vi "HFRR ADV v024 new software.vi"() -> ()   [LabVIEW 2025] (continued)
                  }
                }
              }
            }
          }
        }
        n2655 = case shown="True" w3170 {
          frame False {
            n2656 = local write "tfalg"(0.0 ("tfalg")) -> ()
          }
          frame True {
            n2657 = local read "tfalg"() -> (w3315:dbl)
            n2658 = Equal?(x=w3315, y=0.0) -> (x = y?=w3316:bool)
            n2659 = case shown="True" w3316 {
              frame False {
              }
              frame True {
                n2660 = local read "Total No. of Tests"() -> (w3319:dbl)
                n2661 = local write "tfalg"(1.0 ("tfalg")) -> ()
                n2662 = local write "acq 2"(FALSE ("acq 2")) -> ()
                n2663 = Wait (ms)(milliseconds to wait=u32 200) -> ()  [unwired: 1 out]
                n2664 = Increment(x=w3319) -> (x+1=w3318:dbl)
                n2665 = local write "Total No. of Tests"(w3318) -> ()
              }
            }
          }
        }
        n2666 = local write "Test \nStatus"(w3176) -> ()
        n2667 = local write "Save"(w3176) -> ()
        n2668 = local read "Main Tab"() -> (w3133:T2)
        n2669 = case shown="True" w3157 {
          tunnel: [FALSE ("RUN") TRUE ("RUN")] -> w3156
          tunnel: [_ 1] -> w3149
          frame False {
          }
          frame True {
          }
        }
        n2670 = In Range and Coerce(upper limit=w3164, x=w3137, lower limit=w3163) -> (In Range?=w3155:bool)  [unwired: 1 out]
        n2671 = In Range and Coerce(upper limit=w3161, x=w3136, lower limit=w3162) -> (In Range?=w3153:bool)  [unwired: 1 out]
        n2672 = case shown="True" w3169 {
          frame False {
            n2673 = local read "Rt 3"() -> (w3297:bool)
            n2674 = case shown="True" w3297 {
              frame False {
              }
              frame True {
                n2675 = local write "Rt 3"(FALSE ("Rt 3")) -> ()
                n2676 = local write "Json End Flg"(TRUE ("Upld AR 2")) -> ()
              }
            }
            "Rt" <- TRUE ("Rt")
            "Rt 2" <- FALSE ("Rt")
          }
          frame True {
            n2677 = local read "Rt"() -> (w3304:bool)
            n2678 = local write "Rt 2"(TRUE ("Rt 2")) -> ()
            n2679 = case shown="True" w3304 {
              frame False {
              }
              frame True {
                w3305 = TRUE ("Upld AR 2")
                n2680 = local write "Rt"(FALSE ("Rt")) -> ()
                n2681 = local write "Upld AR"(w3305) -> ()
                n2682 = local write "Json St Flg"(w3305) -> ()
              }
            }
            "Rt 3" <- TRUE ("Rt 3")
          }
        }
        n2683 = case shown="True" w3155 {
          tunnel: [FALSE ("RUN") TRUE ("RUN")] -> w3154
          tunnel: [_ 2] -> w3148
          frame False {
          }
          frame True {
          }
        }
        n2684 = case shown="True" w3153 {
          tunnel: [FALSE ("RUN") TRUE ("RUN")] -> w3152
          tunnel: [_ 3] -> w3147
          frame False {
          }
          frame True {
          }
        }
        n2685 = case shown="\"Acquire\"" w3133 {
          tunnel: w3135 -> [_ w3366]
          frame Default {
            w3365 = 0.0 ("output")
            n2686 = local write "PID-out"(w3365) -> ()
            n2687 = local write "Frequency ( Hz )"(w3365) -> ()
          }
          frame "Acquire" {
            n2688 = stacked-sequence {
              frame #0 {
                n2689 = local read "Auto Start Test"() -> (w3368:bool)
                n2690 = case shown="True" w3368 {
                  tunnel: "RUN" -> [w3389 w3392]
                  tunnel: [w3389 w3391] -> w3369
                  frame False {
                  }
                  frame True {
                    n2691 = local read "Auto Start Temp"() -> (w3390:bool)
                    n2692 = Or(x=w3392, y=w3390) -> (x .or. y?=w3391:bool)
                  }
                }
                n2693 = local read "clk"() -> (w3388:dbl)
                n2694 = local read "Save"() -> (w3384:bool)
                n2695 = Equal?(x=w3388, y=0.0) -> (x = y?=w3385:bool)
                n2696 = And(x=w3385, y=w3384) -> (x .and. y?=w3386:bool)
                n2697 = Not(x="Engage") -> (.not. x?=w3375:bool)
                n2698 = case shown="False" w3369 {
                  tunnel: [0.0 w3415] -> w3371
                  frame False {
                    (unwired) TRUE ("Visible")
                    n2699 = local read "Auto Start Test"() -> (w3396:bool)
                    n2700 = local write "Start Time"(TRUE ("Start Time")) -> ()
                    n2701 = property on="Stroke 2" class="DigNum (strict)"("Visible"=FALSE) -> ()  [unwired: 2 in, 2 out]
                    n2702 = case shown="False" w3396 {
                      frame False {
                        n2703 = property on="Heater Button" class="Bool (strict)"("DisabledEnum"=T19."Enabled" ("Disabled")) -> ()  [unwired: 2 in, 2 out]
                        n2704 = property on="Humidity" class="Bool (strict)"("DisabledEnum"=T19."Enabled" ("Disabled")) -> ()  [unwired: 2 in, 2 out]
                      }
                      frame True {
                      }
                    }
                    n2705 = case shown="False" "TestCompFlg" {
                      frame False {
                        n2706 = local read "StartFlg"() -> (w3404:bool)
                        n2707 = case shown="True" w3404 {
                          frame False {
                          }
                          frame True {
                            n2708 = stacked-sequence {
                              frame #0 {
                                n2709 = local read "EVENT LOG"() -> (w3408:string)
                                n2710 = call "Event Log.vi"("Content"="Test was interrupted", "EVENT LOG"=w3408) -> ("EVENT LOG"=w3409:string)  [unwired: 8 in, 1 out]
                                n2711 = local write "EVENT LOG"(w3409) -> ()
                                n2712 = property on="RUN" class="Bool (strict)"("Visible"=TRUE) -> ()  [unwired: 2 in, 2 out]
                                n2713 = property on="Auto Start Test" class="Bool (strict)"("Visible"=TRUE) -> ()  [unwired: 2 in, 2 out]
                              }
                              frame #1 {
                                w3411 = FALSE ("StartFlg")
                                n2714 = property on="Heater Button" class="Bool (strict)"("Val(Sgnl)"=FALSE ("Value (Signaling)")) -> ()  [unwired: 2 in, 2 out]
                                n2715 = local write "Heater Button"(w3411) -> ()
                                n2716 = local write "StartFlg"(w3411) -> ()
                                n2717 = local write "Humidity"(w3411) -> ()
                              }
                              frame #2 {
                                n2718 = local write "Due Write"("VC;0" ("Command")) -> ()
                              }
                              frame #3 {
                                n2719 = Wait (ms)(milliseconds to wait=u32 1500) -> ()  [unwired: 1 out]
                              }
                              frame #4 {
                                n2720 = local write "Due Write"("HE;0" ("Command")) -> ()
                              }
                            }
                          }
                        }
                      }
                      frame True {
                      }
                    }
                    n2721 = local write "String 14"("Test will autostart once parameters reach the set value." ("String 14")) -> ()
                  }
                  frame True {
                    (unwired) FALSE ("Visible")
                    n2722 = property on="Stroke 2" class="DigNum (strict)"("Visible"=TRUE) -> ()  [unwired: 2 in, 2 out]
                    n2723 = property on="STOP 2" class="Bool (strict)"("Disabled"=u8 2) -> ()  [unwired: 2 in, 2 out]
                    n2724 = local write "String 14"(" Running....." ("String 14")) -> ()
                    n2725 = property on="Heater Button" class="Bool (strict)"("DisabledEnum"=T19."Disabled and Grayed Out" ("Disabled")) -> ()  [unwired: 2 in, 2 out]
                    n2726 = property on="Humidity" class="Bool (strict)"("DisabledEnum"=T19."Disabled and Grayed Out" ("Disabled")) -> ()  [unwired: 2 in, 2 out]
                    n2727 = case shown="True" "Start Time" {
                      selector: "Start Time" -> [_ w3434]
                      frame False {
                      }
                      frame True {
                        n2728 = Not(x=w3434) -> (.not. x?=w3433:bool)
                        n2729 = local write "Start Time"(w3433) -> ()
                        n2730 = local read "EVENT LOG"() -> (w3435:string)
                        n2731 = call "Event Log.vi"("Content"="Test in progress", "EVENT LOG"=w3435) -> ("EVENT LOG"=w3437:string)  [unwired: 8 in, 1 out]
                        n2732 = local write "EVENT LOG"(w3437) -> ()
                      }
                    }
                    n2733 = disable-structure shown="Enabled" {
                      disable-tunnel: [w3426 w3432] -> w3415
                      frame Disabled {
                        n2734 = local read "Set Hz"() -> (w3429:dbl)
                        n2735 = call <vilib>:"Uniform White Noise Waveform.vi"() -> ("signal out"=w3428:waveform(dbl))  [unwired: 10 in, 1 out]
                        n2736 = Random Number (0-1)() -> (number: 0 to 1=w3425:dbl)
                        n2737 = Add(x=w3429, y=w3428) -> (x+y=w3427:waveform(dbl))
                        n2738 = Multiply(x=ext 0.01 ("y"), y=w3425) -> (x*y=w3423:ext)
                        n2739 = Multiply(x=w3427, y=w3423) -> (x*y=w3426:waveform(ext))
                      }
                      frame Enabled {
                        n2740 = call-poly <vilib>:"Random Number (Range).vi"("lower bound (0)"=49.89, "upper bound (100)"=50.8) -> ("number"=w3432:dbl)  [unwired: 9 in]
                      }
                    }
                    "StartFlg" <- TRUE ("StartFlg")
                  }
                }
                n2741 = case shown="True" w3386 {
                  frame False {
                  }
                  frame True {
                    n2742 = local write "clk"(10.0 ("clk")) -> ()
                    n2743 = Get Date/Time In Seconds() -> (seconds since 1Jan1904=w3440:timestamp)
                    n2744 = To Double Precision Float(number=w3440) -> (double precision float=w3438:dbl)
                    n2745 = local write "acq timer"(w3438) -> ()
                    n2746 = local write "act save time"(w3438) -> ()
                  }
                }
                n2747 = call "Elapsed Time"("Time Target (s)"="Countdown", "Reset"=w3375) -> ("Elapsed Time (s)"=w3380:dbl, "Time has Elapsed"=w3378:bool)  [unwired: 10 in, 6 out]
                "Countdown 2" <- w3380
                n2748 = Subtract(x=w3380, y=2.0) -> (x-y=w3383:dbl)
                n2749 = Less?(x=w3383, y="Countdown") -> (x < y?=w3381:bool)
                n2750 = And(x=w3381, y=w3378) -> (x .and. y?=w3377:bool)
                n2751 = case shown="True" w3377 {
                  frame False {
                  }
                  frame True {
                    (unwired) dbl[] [] ("History Data")
                    n2752 = local write "Engage"(FALSE ("Engage")) -> ()
                    n2753 = local write "RUN"(TRUE ("RUN")) -> ()
                    n2754 = local read "Humidity ( %RH )"() -> (→"Rh Before":dbl)
                  }
                }
                n2755 = local read "Test \nStatus"() -> (w3373:bool)
                n2756 = Select(t=w3371, s=w3373, f=0.0) -> (s? t:f=w3372:dbl)
                n2757 = local write "Frequency ( Hz )"(w3372) -> ()
              }
              frame #1 {
                w3463 = 1000000.0 ("x")
                # "HC;1/0\nST;VALUE"
                # "Elapsed time\ncof\nstroke\nAir temp\nTemp\nHumidity"
                # "acq timer\n\nact save time"
                # "convert to microseconds"
                n2758 = local read "COUNT"() -> (w3446:i32)
                n2759 = local read "Rate"() -> (w3459:dbl)
                n2760 = Divide(x=w3463, y=w3459) -> (x/y=w3464:dbl)
                n2761 = Greater Or Equal?(x=w3446, y=250) -> (x >= y?=w3445:bool)
                n2762 = Get Date/Time In Seconds() -> (seconds since 1Jan1904=w3466:timestamp)
                n2763 = case shown="True" w3445 {
                  frame False {
                    n2764 = local read "COUNT"() -> (w3467:i32)
                    n2765 = Increment(x=w3467) -> (x+1=w3468:i32)
                    n2766 = local write "COUNT"(w3468) -> ()
                  }
                  frame True {
                    n2767 = local write "COUNT"(0 ("COUNT")) -> ()
                  }
                }
                n2768 = local read "Samplingtime 2"() -> (w3444:dbl)
                n2769 = local read "act save time"() -> (w3461:dbl)
                n2770 = Divide(x=w3464, y=w3463) -> (x/y=w3462:dbl)
                n2771 = To Double Precision Float(number=w3466) -> (double precision float=w3455:dbl)
                n2772 = Add(x=w3461, y=w3444) -> (x+y=w3460:dbl)
                n2773 = local read "acq timer"() -> (w3465:dbl)
                n2774 = local read "COUNT"() -> (w3448:i32)
                n2775 = Greater Or Equal?(x=w3455, y=w3460) -> (x >= y?=w3443:bool)
                n2776 = Multiply(x=w3462, y=w3448) -> (x*y=w3454:dbl)
                n2777 = Subtract(x=w3455, y=w3465) -> (x-y=w3457:dbl)
                n2778 = local read "Save"() -> (w3458:bool)
                n2779 = Add(x=w3457, y=w3454) -> (x+y=w3441:dbl)
                "Elapsed time 3" <- w3441
                n2780 = And(x=w3443, y=w3458) -> (x .and. y?=w3456:bool)
                n2781 = Divide(x=w3441, y=60.0) -> (x/y=w3452:dbl)
                n2782 = local read "Test \nStatus"() -> (w3442:bool)
                n2783 = local read "clk"() -> (w3449:dbl)
                n2784 = Equal?(x=w3449, y=10.0) -> (x = y?=w3451:bool)
                n2785 = case shown="True" w3456 {
                  tunnel: w3455 -> [_ w3579]
                  tunnel: [FALSE ("Boolean 2") TRUE ("Boolean 2")] -> _
                  frame False {
                  }
                  frame True {
                    w3533 = ";" ("Substring")
                    # "Pid out/\nFreq response value"
                    n2786 = local write "act save time"(w3579) -> ()
                    n2787 = local read "FILE"() -> (w3527:string)
                    n2788 = call "file check.vi"("file name in"=w3527) -> ("error out"=w3530:errorcluster, "file name out"=w3525:string)  [unwired: 9 in]
                    n2789 = local read "LVDT STROKE"() -> (w3522:dbl)
                    n2790 = local read "Add up Stroke"() -> (w3520:dbl)
                    n2791 = call "FILE PATH CREATION.vi"("error in"=w3530, "FILE NAME :"=w3525) -> ("FILE OUT"=w3528:path)  [unwired: 8 in, 1 out]
                    n2792 = Concatenate Strings(w3525, ".dgf" ("Substring")) -> (w3529:string)
                    n2793 = Subtract(x=w3522, y=w3520) -> (x-y=w3521:dbl)
                    n2794 = Absolute Value(x=w3521) -> (abs(x)=w3519:dbl)
                    n2795 = local read "FF 2"() -> (→"Frictional Force ( N )" →"Frictional Force ( N )":dbl)
                    n2796 = Build Path(base path=w3528, name or relative path=w3529) -> (appended path=w3524:path)
                    n2797 = local read "COF 2"() -> (w3538:dbl)
                    "cof" <- w3538
                    "Coefficient of Friction" <- w3538
                    "COF 4" <- w3538
                    "Coefficient of Friction" <- w3538
                    n2798 = local read "TEMP"() -> (w3541:dbl)
                    "Temp" <- w3541
                    "Temperature ( Deg C )" <- w3541
                    n2799 = local read "Humidity ( %RH )"() -> (w3540:dbl)
                    "Humidity ( %RH )" <- w3540
                    "Humidity ( %RH )" <- w3540
                    n2800 = local read "Frequency ( Hz )"() -> (w3547:dbl)
                    n2801 = call <vilib>:"Mean PtByPt.vi"("x"=w3519, "sample length"="STROKE FILTER") -> ("mean"=w3518:dbl)  [unwired: 2 in, 1 out]
                    n2802 = local read "Elapsed time"() -> (w3572:dbl)
                    n2803 = local read "AIR TEMP"() -> (w3545:dbl)
                    n2804 = local read "PID-out"() -> (w3550:dbl)
                    n2805 = local write "Temperature ( Deg C )"(w3541) -> ()
                    n2806 = Number To Fractional String(number=w3518, width (-)=i16 9 ("precision (6)"), precision (6)=i16 6) -> (F-format string=w3565:string)  [unwired: 1 in]
                    n2807 = Number To Fractional String(number=w3545, width (-)=i16 9 ("precision (6)"), precision (6)=i16 3) -> (F-format string=w3564:string)  [unwired: 1 in]
                    n2808 = Number To Fractional String(number=w3541, width (-)=i16 9 ("precision (6)"), precision (6)=i16 3) -> (F-format string=w3561:string)  [unwired: 1 in]
                    n2809 = Number To Fractional String(number=w3540, width (-)=i16 9 ("precision (6)"), precision (6)=i16 3) -> (F-format string=w3558:string)  [unwired: 1 in]
                    n2810 = Number To Fractional String(number=0.0, width (-)=i16 9 ("precision (6)"), precision (6)=i16 3) -> (F-format string=w3555:string)  [unwired: 1 in]
                    n2811 = Number To Fractional String(number=w3550, width (-)=i16 9 ("precision (6)"), precision (6)=i16 3) -> (F-format string=w3551:string)  [unwired: 1 in]
                    n2812 = Number To Fractional String(number=w3547, width (-)=i16 9 ("precision (6)"), precision (6)=i16 3) -> (F-format string=w3546:string)  [unwired: 1 in]
                    n2813 = Number To Fractional String(number=w3538, width (-)=i16 9 ("precision (6)"), precision (6)=i16 6) -> (F-format string=w3573:string)  [unwired: 1 in]
                    n2814 = Number To Fractional String(number=w3572, width (-)=i16 14 ("precision (6)"), precision (6)=i16 3) -> (F-format string=w3574:string)  [unwired: 1 in]
                    n2815 = Bundle("y"=1.02, "mean"=w3518, "y"=0.98) -> (w3539:cluster{"y":dbl, "mean":dbl, "y":dbl})  [unwired: 1 in]
                    n2816 = Number To Fractional String(number="Ambient Humidity :", width (-)=i16 9 ("precision (6)"), precision (6)=i16 6) -> (F-format string=w3531:string)  [unwired: 1 in]
                    n2817 = local read "RUN"() -> (w3537:bool)
                    n2818 = case shown="True" w3537 {
                      tunnel: w3539 -> [_ w3584]
                      tunnel: w3518 -> [_ w3583]
                      tunnel: w3518 -> [_ w3581]
                      tunnel: w3518 -> [_ w3582]
                      frame False {
                      }
                      frame True {
                        "Stroke ( mm )" <- w3584
                        "Stroke ( mm )" <- w3584
                        "Stroke 4" <- w3583
                        "Stroke 3" <- w3581
                        "Stroke 2" <- w3582
                        "measured_stroke" <- w3581
                      }
                    }
                    n2819 = Concatenate Strings(w3574, w3533, w3573, w3533, w3565, w3533, w3564, w3533, w3561, w3533, w3558, w3533, w3555, w3533, w3551, w3533, w3546, w3533, w3531, "\r") -> (w3571:string)
                    n2820 = call <vilib>:"Write Characters To File.vi"("append to file? (new file:F)"=TRUE, "character string"=w3571, "file path (dialog if empty)"=w3524) -> ()  [unwired: 2 in, 1 out]
                    "refresh flag" <- TRUE ("refresh flag")
                  }
                }
                n2821 = case shown="True" w3442 {
                  tunnel: w3452 -> [_ w3478]
                  tunnel: w3457 -> [_ w3488]
                  tunnel: [0.0 w3484] -> _
                  tunnel: w3451 -> [_ w3483]
                  tunnel: [0.0 w3482] -> _
                  tunnel: w3441 -> [_ w3482]
                  tunnel: w3455 -> [w3471 _]
                  frame False {
                    n2822 = local write "acq timer"(w3471) -> ()
                    n2823 = local write "Test Duration Status"(0.0 ("Test Duration Status")) -> ()
                  }
                  frame True {
                    n2824 = local read "Set Hz"() -> (w3485:dbl)
                    n2825 = local write "Elapsed time"(w3478) -> ()
                    n2826 = local read "test time"() -> (w3477:dbl)
                    n2827 = Multiply(x=w3488, y=w3485) -> (x*y=w3487:dbl)
                    n2828 = case shown="False" w3483 {
                      tunnel: w3487 -> [w3489 _]
                      tunnel: [w3489 1.0] -> w3484
                      frame False {
                        n2829 = local write "Cycles elapsed"(w3489) -> ()
                      }
                      frame True {
                      }
                    }
                    n2830 = Greater?(x=w3478, y=w3477) -> (0:w3486:bool)
                    n2831 = Subtract(x=w3477, y=w3478) -> (x-y=w3476:dbl)
                    "time" <- w3476
                    n2832 = Multiply(x=w3476, y=60.0) -> (x*y=w3475:dbl)
                    n2833 = local write "Time Remaining"(w3475) -> ()
                    n2834 = local write "Remaining Time"(w3475) -> ()
                    n2835 = case shown="True" w3486 {
                      frame False {
                      }
                      frame True {
                        n2836 = stacked-sequence {
                          frame #0 {
                            w3494 = T19."Enabled" ("Disabled")
                            w3493 = FALSE ("TEST FILE NAM,E SAVED")
                            w3495 = "" ("FILE")
                            w3496 = TRUE ("Visible")
                            n2837 = local write "Humidity"(FALSE ("Humidity")) -> ()
                            n2838 = local write "RUN"(FALSE ("OK Button 2")) -> ()
                            n2839 = local write "Heater Button"(FALSE ("Heater Button")) -> ()
                            n2840 = local write "Auto Start Test"(FALSE ("Auto Start Test")) -> ()
                            n2841 = local write "TestCompFlg"(TRUE ("StpFlg")) -> ()
                            n2842 = local read "Humidity ( %RH )"() -> (→"Rh After":dbl)
                            n2843 = property on="STOP 2" class="Bool (strict)"("Disabled"=u8 0) -> ()  [unwired: 2 in, 2 out]
                            n2844 = local read "EVENT LOG"() -> (w3501:string)
                            n2845 = call "Event Log.vi"("Content"="Test Completed", "EVENT LOG"=w3501) -> ("EVENT LOG"=w3500:string)  [unwired: 8 in, 1 out]
                            n2846 = property on="RUN" class="Bool (strict)"("Visible"=w3496) -> ()  [unwired: 2 in, 2 out]
                            n2847 = property on="Auto Start Test" class="Bool (strict)"("Visible"=w3496) -> ()  [unwired: 2 in, 2 out]
                            n2848 = local write "Batch Ref Num :"(w3495) -> ()
                            n2849 = local write "FILE"(w3495) -> ()
                            n2850 = local write "EVENT LOG"(w3500) -> ()
                            n2851 = local write "TEST FILE NAM,E SAVED"(w3493) -> ()
                            n2852 = local write "Fuel Discription :"(w3495) -> ()
                            n2853 = local write "START TEMP"(w3493) -> ()
                            n2854 = local write "Remarks :"(w3495) -> ()
                            n2855 = local write "Main Dashboard Buttons"(T1."Imaging" ("Main Dashboard Buttons")) -> ()
                            n2856 = local write "Main Tab"(T2."Adv Scar" ("Main Tab")) -> ()
                            n2857 = property on="FRICVALZ 2" class="Bool (strict)"("DisabledEnum"=w3494) -> ()  [unwired: 2 in, 2 out]
                            n2858 = property on="FRICVALZ 3" class="Bool (strict)"("DisabledEnum"=w3494) -> ()  [unwired: 2 in, 2 out]
                            n2859 = property on="FRICVALZ 4" class="Bool (strict)"("DisabledEnum"=w3494) -> ()  [unwired: 2 in, 2 out]
                          }
                          frame #1 {
                            n2860 = Wait (ms)(milliseconds to wait=u32 1500) -> ()  [unwired: 1 out]
                          }
                          frame #2 {
                            n2861 = local write "Due Write"("VC;0") -> ()
                          }
                          frame #3 {
                            n2862 = Wait (ms)(milliseconds to wait=u32 1500) -> ()  [unwired: 1 out]
                          }
                          frame #4 {
                            n2863 = local write "Due Write"("VC;0") -> ()
                          }
                          frame #5 {
                            n2864 = Wait (ms)(milliseconds to wait=u32 1500) -> ()  [unwired: 1 out]
                          }
                          frame #6 {
                            n2865 = local write "Due Write"("ST;0") -> ()
                          }
                          frame #7 {
                            n2866 = local write "measured_stroke"(0.0 ("measured_stroke")) -> ()
                            n2867 = Wait (ms)(milliseconds to wait=u32 1500) -> ()  [unwired: 1 out]
                          }
                          frame #8 {
                            n2868 = local write "Due Write"("HE;0") -> ()
                          }
                        }
                      }
                    }
                    n2869 = Divide(x=w3478, y=w3477) -> (x/y=w3481:dbl)
                    n2870 = Multiply(x=w3481, y=100.0) -> (x*y=w3479:dbl)
                    n2871 = local write "Test Duration Status"(w3479) -> ()
                  }
                }
              }
              frame #2 {
                n2872 = case shown="True" "Heater Button" {
                  tunnel: [0.0 ("output") w3607] -> w3585
                  frame False {
                    w3588 = TRUE ("tmpchk")
                    n2873 = local read "TEMP"() -> (w3589:dbl)
                    n2874 = local write "Temp ini"(w3589) -> ()
                    n2875 = local write "Reset 4"(w3588) -> ()
                    n2876 = local write "tmpchk"(w3588) -> ()
                    n2877 = local write "reinit"(TRUE ("reinit")) -> ()
                    n2878 = local write "manual temp log"(TRUE ("manual temp log")) -> ()
                  }
                  frame True {
                    # "Logic to turn off\nthe heater when \ntemp is not rising.\nTime - 60 sec\nDelta t- 5°c"
                    n2879 = local read "Temp ini"() -> (w3596:dbl)
                    n2880 = local read "Auto Start Test"() -> (w3592:bool)
                    n2881 = Less?(x=w3596, y=53.0) -> (x < y?=w3594:bool)
                    n2882 = case shown="False" w3592 {
                      frame False {
                        n2883 = local read "Set Temp"() -> (w3616:dbl)
                        n2884 = local read "TEMP"() -> (w3615:dbl)
                        n2885 = Subtract(x=w3616, y=w3615) -> (x-y=w3614:dbl)
                        n2886 = Absolute Value(x=w3614) -> (abs(x)=w3613:dbl)
                        n2887 = Less?(x=w3613, y=0.5) -> (x < y?=w3611:bool)
                        n2888 = case shown="True" w3611 {
                          tunnel: "manual temp log" -> [_ w3617]
                          frame False {
                          }
                          frame True {
                            n2889 = case shown="True" w3617 {
                              selector: w3617 -> [_ w3618]
                              frame False {
                              }
                              frame True {
                                # "#Event log"
                                n2890 = Not(x=w3618) -> (.not. x?=w3619:bool)
                                n2891 = local write "manual temp log"(w3619) -> ()
                                n2892 = local read "EVENT LOG"() -> (w3622:string)
                                n2893 = call "Event Log.vi"("Content"="Target Temperature reached", "EVENT LOG"=w3622) -> ("EVENT LOG"=w3621:string)  [unwired: 8 in, 1 out]
                                n2894 = local write "EVENT LOG"(w3621) -> ()
                              }
                            }
                          }
                        }
                      }
                      frame True {
                        n2895 = local write "manual temp log"(TRUE ("manual temp log")) -> ()
                      }
                    }
                    n2896 = And(x="tmpchk", y=w3594) -> (x .and. y?=w3597:bool)
                    n2897 = case shown="True" w3597 {
                      frame False {
                      }
                      frame True {
                        n2898 = call "Elapsed Time8"("Time Target (s)"=300.0, "Reset"="Reset 4") -> ("Time has Elapsed"=w3624:bool)  [unwired: 10 in, 7 out]
                        n2899 = flat-sequence {
                          tunnel: w3624 -> [_]
                          frame #0 {
                            n2900 = local write "Reset 4"(FALSE ("Reset 4")) -> ()
                          }
                        }
                        n2901 = case shown="True" w3624 {
                          frame False {
                          }
                          frame True {
                            n2902 = local read "Temp ini"() -> (w3631:dbl)
                            n2903 = Add(x=w3631, y=5.0) -> (x+y=w3629:dbl)
                            n2904 = local read "TEMP"() -> (w3632:dbl)
                            n2905 = Greater?(x=w3632, y=w3629) -> (0:w3630:bool)
                            n2906 = case shown="False" w3630 {
                              frame False {
                                n2907 = local write "Heater Button"(FALSE ("Heater Button")) -> ()
                              }
                              frame True {
                                n2908 = local write "tmpchk"(FALSE ("tmpchk")) -> ()
                              }
                            }
                          }
                        }
                      }
                    }
                    n2909 = local read "Set Temp"() -> (w3605:dbl)
                    n2910 = local read "TEMP"() -> (w3599:dbl)
                    n2911 = call-poly <vilib>:"PID.vi"("reinitialize? (F)"="reinit", "dt (s)"=-1.0, "process variable"=w3599, "setpoint"=w3605) -> ("output"=w3602:dbl)  [unwired: 6 in, 1 out]
                    n2912 = Subtract(x=w3605, y=w3599) -> (x-y=w3606:dbl)
                    n2913 = Add(x=w3605, y=0.5) -> (x+y=w3603:dbl)
                    n2914 = Greater Or Equal?(x=w3599, y=w3603) -> ()  [unwired: 1 out]
                    n2915 = Select(t=0.0, s=FALSE, f=w3602) -> (s? t:f=w3601:dbl)
                    "PID output" <- w3601
                    n2916 = flat-sequence {
                      tunnel: w3601 -> [w3635]
                      tunnel: [w3635] -> w3607
                      frame #0 {
                        n2917 = local write "reinit"(FALSE ("reinit")) -> ()
                      }
                    }
                    n2918 = Bundle(w3606, "output"=w3601, "TEMP"=w3599) -> ()  [unwired: 1 in, 1 out]
                  }
                }
                "PID-out" <- w3585
              }
              frame #3 {
                n2919 = local read "TEMP"() -> (w3637:dbl)
                n2920 = Greater Or Equal?(x=w3637, y="Set Temp 2") -> (x >= y?=w3642:bool)
                n2921 = case shown="True" w3642 {
                  tunnel: [FALSE TRUE] -> w3640
                  frame False {
                  }
                  frame True {
                  }
                }
                "Status 13" <- w3640
                n2922 = And(x=w3640, y="trip1 8") -> (x .and. y?=w3639:bool)
                n2923 = case shown="True" w3639 {
                  frame False {
                    n2924 = local write "Heater Trip Temp"(TRUE ("Heater Trip Temp")) -> ()
                  }
                  frame True {
                    w3645 = FALSE ("OK Button 2")
                    n2925 = case shown="True" "Heater Trip Temp" {
                      selector: "Heater Trip Temp" -> [_ w3647]
                      frame False {
                      }
                      frame True {
                        n2926 = Not(x=w3647) -> (.not. x?=w3646:bool)
                        n2927 = local read "EVENT LOG"() -> (w3650:string)
                        n2928 = local write "Heater Trip Temp"(w3646) -> ()
                        n2929 = call "Event Log.vi"("Content"="Heater Trip", "EVENT LOG"=w3650) -> ("EVENT LOG"=w3649:string)  [unwired: 8 in, 1 out]
                        n2930 = local write "EVENT LOG"(w3649) -> ()
                      }
                    }
                    n2931 = local write "RUN"(w3645) -> ()
                    n2932 = property on="Auto Start Test" class="Bool (strict)"("Value"=w3645) -> ()  [unwired: 2 in, 2 out]
                    n2933 = local write "Heater Button"(w3645) -> ()
                  }
                }
              }
            }
            n2934 = case shown="False" w3366 {
              frame False {
                n2935 = disable-structure shown="Disabled" {
                  frame Disabled {
                    n2936 = stacked-sequence {
                      frame #0 {
                        n2937 = local write "RUN"(FALSE ("OK Button 2")) -> ()
                      }
                      frame #1 {
                      }
                    }
                  }
                  frame Enabled {
                  }
                }
              }
              frame True {
              }
            }
          }
        }
        n2938 = local read "airtempflg"() -> (w3158:bool)
        n2939 = Or(x=w3158, y=w3156) -> (x .or. y?=w3159:bool)
        n2940 = Insert Into Array(array=string[] ["Air Temperature has reached set value,", "Humidity has reached set value,", "Sample Temperaturehas reached set value,", ""], index=0, new element="") -> (w3144:string[])
        n2941 = Build Array(w3149, w3148, w3147) -> (w3145:i32[])
        n2942 = disable-structure shown="Disabled" {
          disable-tunnel: w3159 -> [w3236 _]
          disable-tunnel: w3154 -> [w3235 _]
          disable-tunnel: w3152 -> [w3234 _]
          frame Disabled {
            n2943 = Compound Arithmetic op=AND(w3236, w3235, w3234) -> ()  [unwired: 1 out]
            n2944 = case shown="True" {
              selector: _ -> [_ _]
              frame False {
              }
              frame True {
                w3237 = FALSE ("autostrtflg")
                n2945 = local write "RUN"(TRUE ("RUN")) -> ()
                n2946 = local write "autostrtflg"(w3237) -> ()
                n2947 = local write "autostart"(w3237) -> ()
                n2948 = local write "String 14"(" Running....." ("String 14")) -> ()
              }
            }
          }
          frame Enabled {
          }
        }
        n2949 = for {
          tunnel: w3145 -> [w3287] mode=indexing
          tunnel: w3144 -> [w3286]
          shift-right: [w3283] -> w3143
          shift-left: "" -> [w3285]
          n2950 = Index Array(array=w3286, index=w3287) -> (element=w3284:string)
          n2951 = Concatenate Strings(w3284, w3285) -> (w3283:string)
        }
        n2952 = local write "autostart 2"(w3143) -> ()
        n2953 = local read "Reset Graph"() -> (w3132:bool)
        n2954 = case shown="True" w3132 {
          selector: w3132 -> [_ w3186]
          frame False {
          }
          frame True {
            w3200 = 0.0 ("X Scale.Range:Maximum")
            n2955 = Not(x=w3186) -> (.not. x?=w3185:bool)
            n2956 = local write "Reset Graph"(w3185) -> ()
            n2957 = property on="Electrical Contact Resistance ( % )" class="WFChart (strict)"("XScale.Maximum"=600.0 ("X Scale.Range:Maximum"), "XScale.Minimum"=0.0 ("X Scale.Range:Minimum"), "YScale.Maximum"=100.0 ("Y Scale.Range:Maximum"), "YScale.Minimum"=0.0 ("Y Scale.Range:Minimum")) -> ()  [unwired: 2 in, 2 out]
            n2958 = property on="Frictional Force ( N )" class="WFChart (strict)"("XScale.Maximum"=600.0 ("X Scale.Range:Maximum"), "XScale.Minimum"=0.0 ("X Scale.Range:Minimum"), "YScale.Maximum"=100.0 ("Y Scale.Range:Maximum"), "YScale.Minimum"=0.0 ("Y Scale.Range:Minimum")) -> ()  [unwired: 2 in, 2 out]
            n2959 = property on="Temperature ( Deg C )" class="WFChart (strict)"("XScale.Maximum"=600.0 ("X Scale.Range:Maximum"), "XScale.Minimum"=0.0 ("X Scale.Range:Minimum"), "YScale.Maximum"=100.0 ("Y Scale.Range:Maximum"), "YScale.Minimum"=0.0 ("Y Scale.Range:Minimum")) -> ()  [unwired: 2 in, 2 out]
            n2960 = property on="Humidity ( %RH )" class="WFChart (strict)"("XScale.Maximum"=600.0 ("X Scale.Range:Maximum"), "XScale.Minimum"=0.0 ("X Scale.Range:Minimum"), "YScale.Maximum"=100.0 ("Y Scale.Range:Maximum"), "YScale.Minimum"=0.0 ("Y Scale.Range:Minimum")) -> ()  [unwired: 2 in, 2 out]
            n2961 = property on="Stroke ( mm )" class="WFChart (strict)"("XScale.Maximum"=600.0 ("X Scale.Range:Maximum"), "XScale.Minimum"=0.0 ("X Scale.Range:Minimum"), "YScale.Maximum"=100.0 ("Y Scale.Range:Maximum"), "YScale.Minimum"=0.0 ("Y Scale.Range:Minimum")) -> ()  [unwired: 2 in, 2 out]
            n2962 = property on="Coefficient of Friction" class="WFChart (strict)"("XScale.Maximum"=600.0 ("X Scale.Range:Maximum"), "XScale.Minimum"=0.0 ("X Scale.Range:Minimum"), "YScale.Maximum"=100.0 ("Y Scale.Range:Maximum"), "YScale.Minimum"=0.0 ("Y Scale.Range:Minimum")) -> ()  [unwired: 2 in, 2 out]
            n2963 = property on="Electrical Contact Resistance ( % )" class="WFChart (strict)"("XScale.Minimum"=0.0 ("X Scale.Range:Minimum"), "XScale.Maximum"=600.0 ("X Scale.Range:Maximum"), "YScale.Minimum"=0.0 ("Y Scale.Range:Minimum"), "YScale.Maximum"=100.0 ("Y Scale.Range:Maximum")) -> ()  [unwired: 2 in, 2 out]
            n2964 = property on="Temperature ( Deg C )" class="WFChart (strict)"("XScale.Minimum"=0.0 ("X Scale.Range:Minimum"), "XScale.Maximum"=600.0 ("X Scale.Range:Maximum"), "YScale.Minimum"=0.0 ("Y Scale.Range:Minimum"), "YScale.Maximum"=100.0 ("Y Scale.Range:Maximum")) -> ()  [unwired: 2 in, 2 out]
            n2965 = property on="Coefficient of Friction" class="WFChart (strict)"("XScale.Minimum"=0.0 ("X Scale.Range:Minimum"), "XScale.Maximum"=600.0 ("X Scale.Range:Maximum"), "YScale.Maximum"=1.0 ("X Scale.Range:Minimum"), "YScale.Minimum"=0.0 ("X Scale.Range:Minimum")) -> ()  [unwired: 2 in, 2 out]
            n2966 = property on="Frictional Force ( N )" class="WFChart (strict)"("XScale.Maximum"=600.0 ("X Scale.Range:Maximum"), "XScale.Minimum"=w3200, "YScale.Maximum"=10.0 ("Y Scale.Range:Maximum"), "YScale.Minimum"=w3200) -> ()  [unwired: 2 in, 2 out]
            n2967 = property on="Stroke ( mm )" class="WFChart (strict)"("XScale.Maximum"=600.0 ("X Scale.Range:Maximum"), "XScale.Minimum"=0.0 ("X Scale.Range:Minimum"), "YScale.Maximum"=100.0 ("Y Scale.Range:Maximum"), "YScale.Minimum"=0.0 ("Y Scale.Range:Minimum")) -> ()  [unwired: 2 in, 2 out]
            n2968 = property on="Humidity ( %RH )" class="WFChart (strict)"("XScale.Maximum"=600.0 ("X Scale.Range:Maximum"), "XScale.Minimum"=0.0 ("X Scale.Range:Minimum"), "YScale.Maximum"=100.0 ("Y Scale.Range:Maximum"), "YScale.Minimum"=0.0 ("Y Scale.Range:Minimum")) -> ()  [unwired: 2 in, 2 out]
          }
        }
      }
      frame "Compare Files" {
        # "Elapsed time\ncof\nstroke\nAir temp\nTemp\nHumidity"
        n2969 = case shown="True" "RSTV1 2" {
          frame False {
          }
          frame True {
            n2970 = property on="Humidity ( %RH )" class="XYGraph (strict)"("Y Scale.Display Format:Precision"=u8 0 ("Y Scale.Format & Precision:Precision")) -> ()  [unwired: 2 in, 2 out]
            n2971 = property on="Humidity ( %RH )" class="XYGraph (strict)"("X Scale.Range:Minimum"=0.0, "X Scale.Range:Maximum"=75.0, "Y Scale.Range:Minimum"=48.0, "Y Scale.Range:Maximum"=58.0) -> ()  [unwired: 2 in, 2 out]
          }
        }
        n2972 = case shown="True" "RST CP 2" {
          frame False {
          }
          frame True {
            n2973 = property on="XY Graph 13" class="XYGraph (strict)"("Y Scale.Display Format:Precision"=u8 0 ("Y Scale.Format & Precision:Precision")) -> ()  [unwired: 2 in, 2 out]
            n2974 = property on="XY Graph 13" class="XYGraph (strict)"("X Scale.Range:Minimum"=0.0, "X Scale.Range:Maximum"=75.0, "Y Scale.Range:Minimum"=0.0, "Y Scale.Range:Maximum"=100.0) -> ()  [unwired: 2 in, 2 out]
          }
        }
        n2975 = case shown="True" "RST CP" {
          frame False {
          }
          frame True {
            n2976 = property on="Sample Temperature ( °C )" class="XYGraph (strict)"("Y Scale.Display Format:Precision"=u8 2 ("Y Scale.Format & Precision:Precision")) -> ()  [unwired: 2 in, 2 out]
            n2977 = property on="Sample Temperature ( °C )" class="XYGraph (strict)"("X Scale.Range:Minimum"=0.0, "X Scale.Range:Maximum"=75.0, "Y Scale.Range:Minimum"=58.0, "Y Scale.Range:Maximum"=62.0) -> ()  [unwired: 2 in, 2 out]
          }
        }
        n2978 = case shown="True" "RSTV1 3" {
          frame False {
          }
          frame True {
            n2979 = property on="Air Temperature  ( °C )" class="XYGraph (strict)"("Y Scale.Display Format:Precision"=u8 2 ("Y Scale.Format & Precision:Precision")) -> ()  [unwired: 2 in, 2 out]
            n2980 = property on="Air Temperature  ( °C )" class="XYGraph (strict)"("X Scale.Range:Minimum"=0.0 ("Y Scale.Range:Minimum"), "X Scale.Range:Maximum"=75.0 ("Y Scale.Range:Maximum"), "Y Scale.Range:Minimum"=20.0 ("X Scale.Range:Minimum"), "Y Scale.Range:Maximum"=26.0 ("X Scale.Range:Maximum")) -> ()  [unwired: 2 in, 2 out]
          }
        }
        n2981 = case shown="True" "RSTV1 4" {
          frame False {
          }
          frame True {
            n2982 = property on="Stroke ( mm )" class="XYGraph (strict)"("Y Scale.Display Format:Precision"=u8 2 ("Y Scale.Format & Precision:Precision")) -> ()  [unwired: 2 in, 2 out]
            n2983 = property on="Stroke ( mm )" class="XYGraph (strict)"("X Scale.Range:Minimum"=0.0 ("Y Scale.Range:Maximum"), "X Scale.Range:Maximum"=75.0 ("X Scale.Range:Minimum"), "Y Scale.Range:Minimum"=0.98, "Y Scale.Range:Maximum"=1.02) -> ()  [unwired: 2 in, 2 out]
          }
        }
        n2984 = case shown="True" "rstv2" {
          frame False {
          }
          frame True {
            n2985 = property on="Coefficient Of Friction" class="XYGraph (strict)"("Y Scale.Display Format:Precision"=u8 3 ("Y Scale.Format & Precision:Precision")) -> ()  [unwired: 2 in, 2 out]
            n2986 = property on="Coefficient Of Friction" class="XYGraph (strict)"("X Scale.Range:Minimum"=0.0 ("Y Scale.Range:Maximum"), "X Scale.Range:Maximum"=75.0, "Y Scale.Range:Minimum"=0.0, "Y Scale.Range:Maximum"=1.0 ("X Scale.Range:Minimum")) -> ()  [unwired: 2 in, 2 out]
          }
        }
        n2987 = case shown="True" "RST CP 3" {
          frame False {
          }
          frame True {
            n2988 = property on="Air Temp ( °C ) vs Humidity ( % RH )" class="XYGraph (strict)"("X Scale.Range:Minimum"=18.0, "X Scale.Range:Maximum"=28.0 ("X Scale.Range:Minimum"), "Y Scale.Range:Minimum"=30.0 ("X Scale.Range:Minimum"), "Y Scale.Range:Maximum"=70.0 ("X Scale.Range:Minimum")) -> ()  [unwired: 2 in, 2 out]
          }
        }
        n2989 = case shown="True" "OPEN 1" {
          frame False {
          }
          frame True {
            (unwired) 0  # existing file
            w3926 = "Choose a datalog file to open"  # prompt
            n2990 = local write "OPEN 1"(FALSE ("OPEN 1")) -> ()
            n2991 = String To Path(string="C:\\LAB-IQ\\Data\\") -> (path=w3911:path)
            n2992 = File Dialog(6:"*.dgf" ("pattern"), 7:w3926, 11:w3911) -> (0:w3909:errorcluster, 3:w3917:path)  [unwired: 4 in, 2 out]
            n2993 = Unbundle(w3909) -> ()  [unwired: 3 out]
            n2994 = Strip Path(path=w3917) -> (name=w3916:string)  [unwired: 1 out]
            n2995 = Path To String(path=w3917) -> (string=w3912:string)
            "string1" <- w3912
            n2996 = Match Pattern(string=w3916, regular expression=".dgf") -> (before substring=→"String Control":string)  [unwired: 1 in, 3 out]
            n2997 = Match Pattern(string=w3912, regular expression=".dgf" ("substring (\"\")")) -> (before substring=w3922:string)  [unwired: 1 in, 3 out]
            n2998 = Concatenate Strings(w3922, ".duf" ("Substring")) -> (w3918:string)
            n2999 = String To Path(string=w3918) -> (path=w3923:path)
            n3000 = call <vilib>:"Read Characters From File.vi"("file path (dialog if empty)"=w3923, "start of read offset (chars.:0)"=60 ("start of read offset (chars.: 0)")) -> ("character string"=→"String Control 2":string)  [unwired: 4 in, 3 out]
          }
        }
        n3001 = case shown="True" "OPEN 2" {
          frame False {
          }
          frame True {
            (unwired) 0  # existing file
            w3944 = "Choose a datalog file to open"  # prompt
            n3002 = local write "OPEN 2"(FALSE ("OPEN 1")) -> ()
            n3003 = String To Path(string="C:\\LAB-IQ\\Data\\") -> (path=w3929:path)
            n3004 = File Dialog(6:"*.dgf" ("pattern"), 7:w3944, 11:w3929) -> (0:w3927:errorcluster, 3:w3935:path)  [unwired: 4 in, 2 out]
            n3005 = Unbundle(w3927) -> ()  [unwired: 3 out]
            n3006 = Strip Path(path=w3935) -> (name=w3933:string)  [unwired: 1 out]
            n3007 = Path To String(path=w3935) -> (string=w3930:string)
            "string1 2" <- w3930
            n3008 = Match Pattern(string=w3933, regular expression=".dgf") -> (before substring=→"String Control 3":string)  [unwired: 1 in, 3 out]
            n3009 = Match Pattern(string=w3930, regular expression=".dgf" ("substring (\"\")")) -> (before substring=w3941:string)  [unwired: 1 in, 3 out]
            n3010 = Concatenate Strings(w3941, ".duf" ("Substring")) -> (w3938:string)
            n3011 = String To Path(string=w3938) -> (path=w3936:path)
            n3012 = call <vilib>:"Read Characters From File.vi"("file path (dialog if empty)"=w3936, "start of read offset (chars.:0)"=60 ("start of read offset (chars.: 0)")) -> ("character string"=→"String Control 4":string)  [unwired: 4 in, 3 out]
          }
        }
        n3013 = case shown="True" "OPEN 3" {
          frame False {
          }
          frame True {
            (unwired) 0  # existing file
            w3962 = "Choose a datalog file to open"  # prompt
            n3014 = local write "OPEN 3"(FALSE ("OPEN 1")) -> ()
            n3015 = String To Path(string="C:\\LAB-IQ\\Data\\") -> (path=w3947:path)
            n3016 = File Dialog(6:"*.dgf" ("pattern"), 7:w3962, 11:w3947) -> (0:w3945:errorcluster, 3:w3953:path)  [unwired: 4 in, 2 out]
            n3017 = Unbundle(w3945) -> ()  [unwired: 3 out]
            n3018 = Strip Path(path=w3953) -> (name=w3951:string)  [unwired: 1 out]
            n3019 = Path To String(path=w3953) -> (string=w3948:string)
            "string1 3" <- w3948
            n3020 = Match Pattern(string=w3951, regular expression=".dgf") -> (before substring=→"String Control 5":string)  [unwired: 1 in, 3 out]
            n3021 = Match Pattern(string=w3948, regular expression=".dgf" ("substring (\"\")")) -> (before substring=w3958:string)  [unwired: 1 in, 3 out]
            n3022 = Concatenate Strings(w3958, ".duf" ("Substring")) -> (w3955:string)
            n3023 = String To Path(string=w3955) -> (path=w3959:path)
            n3024 = call <vilib>:"Read Characters From File.vi"("file path (dialog if empty)"=w3959, "start of read offset (chars.:0)"=60 ("start of read offset (chars.: 0)")) -> ("character string"=→"String Control 6":string)  [unwired: 4 in, 3 out]
          }
        }
        n3025 = case shown="True" "OPEN 4" {
          frame False {
          }
          frame True {
            (unwired) 0  # existing file
            w3980 = "Choose a datalog file to open"  # prompt
            n3026 = local write "OPEN 4"(FALSE ("OPEN 1")) -> ()
            n3027 = String To Path(string="C:\\LAB-IQ\\Data\\") -> (path=w3965:path)
            n3028 = File Dialog(6:"*.dgf" ("pattern"), 7:w3980, 11:w3965) -> (0:w3963:errorcluster, 3:w3971:path)  [unwired: 4 in, 2 out]
            n3029 = Unbundle(w3963) -> ()  [unwired: 3 out]
            n3030 = Strip Path(path=w3971) -> (name=w3969:string)  [unwired: 1 out]
            n3031 = Path To String(path=w3971) -> (string=w3966:string)
            "string1 4" <- w3966
            n3032 = Match Pattern(string=w3969, regular expression=".dgf") -> (before substring=→"String Control 7":string)  [unwired: 1 in, 3 out]
            n3033 = Match Pattern(string=w3966, regular expression=".dgf" ("substring (\"\")")) -> (before substring=w3976:string)  [unwired: 1 in, 3 out]
            n3034 = Concatenate Strings(w3976, ".duf" ("Substring")) -> (w3973:string)
            n3035 = String To Path(string=w3973) -> (path=w3977:path)
            n3036 = call <vilib>:"Read Characters From File.vi"("file path (dialog if empty)"=w3977, "start of read offset (chars.:0)"=60 ("start of read offset (chars.: 0)")) -> ("character string"=→"String Control 8":string)  [unwired: 4 in, 3 out]
          }
        }
      }
      frame "About" {
        # "Elapsed time\ncof\nstroke\nmean pos\nTemp\nHumidity"
        n3037 = disable-structure shown="Disabled" {
          frame Disabled {
            n3038 = case shown="True" "Export" {
              frame False {
              }
              frame True {
                w4002 = "                                      " ("string")
                w4004 = "\r"
                (unwired) i16 6 ("width (-)")
                w4081 = "\r"
                w4013 = "\r"
                n3039 = local write "Export"(FALSE ("Export")) -> ()
                n3040 = local read "String 29"() -> (w4050:string)
                n3041 = local read "String 34"() -> (w4038:string)
                n3042 = local read "String 35"() -> (w4033:string)
                n3043 = local read "String 37"() -> (w4029:string)
                n3044 = local read "String 36"() -> (w4026:string)
                n3045 = local read "String 38"() -> (w4023:string)
                n3046 = local read "String 39"() -> (w4020:string)
                n3047 = Match Pattern(string=w4050, regular expression=".dwm") -> (before substring=w4046:string)  [unwired: 1 in, 3 out]
                "before substring" <- w4046
                n3048 = local read "S 38"() -> (w4041:string)
                n3049 = local read "S 39"() -> (w4034:string)
                n3050 = local read "Temperature before test 2"() -> (w4070:dbl)
                n3051 = local read "Temperature after test 2"() -> (w4075:dbl)
                n3052 = local read "Humidity before test 2"() -> (w4056:dbl)
                n3053 = local read "Humidity after test 2"() -> (w4071:dbl)
                n3054 = local read "MWSD 2"() -> (w4067:dbl)
                n3055 = local read "WS1.4 2"() -> (w4083:dbl)
                n3056 = local read "HCF 2"() -> (w4079:dbl)
                n3057 = local read "AVP 2"() -> (w4068:dbl)
                n3058 = Concatenate Strings("1," ("string"), w4041) -> (w4040:string)
                n3059 = Concatenate Strings("2," ("string"), w4038) -> (w4037:string)
                n3060 = Concatenate Strings("3," ("string"), w4034) -> (w4036:string)
                n3061 = Concatenate Strings("4," ("string"), w4033) -> (w4032:string)
                n3062 = Concatenate Strings("5," ("string"), w4029) -> (w4030:string)
                n3063 = Concatenate Strings("6," ("string"), w4026) -> (w4027:string)
                n3064 = Concatenate Strings("7," ("string"), w4023) -> (w4024:string)
                n3065 = Concatenate Strings("8," ("string"), w4020) -> (w4021:string)
                n3066 = local read "Sample ID"() -> (w4088:string)
                n3067 = case shown="\"xlx\"" "Select File Type" {
                  tunnel: w4046 -> [w4091 w4093 w4095]
                  tunnel: [w4089 w4094 w4096] -> w4045
                  frame "xlx" {
                    n3068 = Concatenate Strings(w4091, ".xls" ("string")) -> (w4089:string)
                  }
                  frame "csv" {
                    n3069 = Concatenate Strings(w4093, ".csv" ("string")) -> (w4094:string)
                  }
                  frame "txt" {
                    n3070 = Concatenate Strings(w4095, ".txt" ("string")) -> (w4096:string)
                  }
                }
                n3071 = local read "Test Date"() -> (w4087:string)
                n3072 = local read "String 45"() -> (w4001:string)
                n3073 = local read "String 31"() -> (w4086:string)
                n3074 = local read "String 32"() -> (w4085:string)
                n3075 = local read "TITTLE"() -> (w4009:string)
                n3076 = Number To Fractional String(number=w4056, width (-)=i16 6, precision (6)=i16 2) -> (F-format string=w4055:string)  [unwired: 1 in]
                n3077 = Number To Fractional String(number=w4070, width (-)=i16 6, precision (6)=i16 2) -> (F-format string=w4076:string)  [unwired: 1 in]
                n3078 = Number To Fractional String(number=w4071, width (-)=i16 6, precision (6)=i16 2) -> (F-format string=w4069:string)  [unwired: 1 in]
                n3079 = Number To Fractional String(number=w4075, width (-)=i16 6, precision (6)=i16 2) -> (F-format string=w4074:string)  [unwired: 1 in]
                n3080 = Number To Fractional String(number=w4067, width (-)=i16 6, precision (6)=i16 2) -> (F-format string=w4065:string)  [unwired: 1 in]
                n3081 = Number To Fractional String(number=w4068, width (-)=i16 6, precision (6)=i16 2) -> (F-format string=w4066:string)  [unwired: 1 in]
                n3082 = Number To Fractional String(number=w4079, width (-)=i16 6, precision (6)=i16 2) -> (F-format string=w4080:string)  [unwired: 1 in]
                n3083 = Number To Fractional String(number=w4083, precision (6)=i16 2) -> (F-format string=w4084:string)  [unwired: 2 in]
                n3084 = local read "s.NO"() -> (w4003:string)
                n3085 = Concatenate Strings("=" ("string"), w4009) -> (w4008:string)
                n3086 = Concatenate Strings("S.No," ("string"), "                                       Parameters" ("string")) -> (w4014:string)
                n3087 = Concatenate Strings(w4081, w4040, w4055, w4081, w4037, w4076, w4081, w4036, w4069, w4081, w4032, w4074, w4081, w4030, w4065, w4081, w4027, w4066, w4081, w4024, w4080, w4081, w4021, w4084) -> (w4043:string)
                n3088 = Concatenate Strings(w4013, "," ("string"), w4001, w4003, w4002, w4085, w4088, w4002, w4086, w4087, w4013) -> (w4011:string)
                n3089 = local read "Tested by"() -> (w4017:string)
                n3090 = local read "String 33"() -> (w4018:string)
                n3091 = Concatenate Strings("," ("string"), "                                                                             " ("string")) -> (w4006:string)
                n3092 = Concatenate Strings(w4008, w4004, w4011, w4004, w4014, w4043, w4004, w4006, w4018, w4017) -> (→"export":string)
                n3093 = String To Path(string=w4045) -> (path=w4052:path)
                n3094 = local read "export"() -> (w4047:string)
                n3095 = call <vilib>:"Write Characters To File.vi"("append to file? (new file:F)"=FALSE, "character string"=w4047, "file path (dialog if empty)"=w4052) -> ()  [unwired: 2 in, 1 out]
              }
            }
          }
          frame Enabled {
          }
        }
        n3096 = case shown="True" "OK Button 17" {
          frame False {
          }
          frame True {
            (unwired) 0  # existing file
            w4305 = "Choose a datalog file to open"  # prompt
